vi "Read_Temp.vi"() -> ()   [LabVIEW 2013]
uses:
  <instrlib>/Mercury iXX/Public/Controls/Comms Transport Layer.ctl
  <instrlib>/Mercury iXX/Public/Controls/Serial Settings.ctl
  <instrlib>/Mercury iXX/Public/Controls/ISOBus Address.ctl
  <instrlib>/Mercury iXX/Public/Controls/Unit String.ctl
  <instrlib>/Mercury iXX/Public/Libraries/System/Open/Open System.vi
  <instrlib>/Mercury iXX/Public/Libraries/System/Read/Catalogue (Read).vi
  <instrlib>/Mercury iXX/Public/Libraries/Temperature/Open/Open Temperature Device.vi
  <instrlib>/Mercury iXX/Public/Libraries/Temperature/Signals/Read/Temperature (Read).vi
  <instrlib>/Mercury iXX/Mercury iXX.lvlib
  <instrlib>/Mercury iXX/Public/Libraries/System.lvlib
  <instrlib>/Mercury iXX/Public/Libraries/Temperature.lvlib
panel:
  in  "Read Interval (s)":sgl=1.0 min=0.25 max=1000 step=0.25 format="%.2f"
  in  "stop":bool
  out "Unit":T1
  out "Temperature":dbl
  out "error out":errorcluster
  in  "Device Identifier":string="MB1.T1:TEMP"
  in  "ISOBUS address":T2=-1 caption="ISOBUS address (-1)"
  out "Devices":string[](array[string])
  in  "Clear Previous Connections (False)":bool
  in  "ID Query (True)":bool
  in  "Serial Configuration":T3={"Baud Rate"=9600, "Parity"=0, "Data Bits"=8, "Stop Bits"=10, "Flow Control"=0} {"Flow Control" items=["None", "XON/XOFF", "RTS/CTS", "XON/XOFF & RTS/CTS", "DTR/DSR", "XON/XOFF & DTR/DSR"]; "Stop Bits" items=["1.0"=10, "2.0"=20]; "Data Bits" items=["7"=7, "8"=8]; "Parity" items=["None", "Odd", "Even"]; "Baud Rate" items=["300"=300, "600"=600, "1200"=1200, "2400"=2400, "4800"=4800, "9600"=9600, "19200"=19200]}
  in  "Comms Layer":T4
  in  "IP Address":string
  in  "VISA resource name":refnum<visa-resource-name>
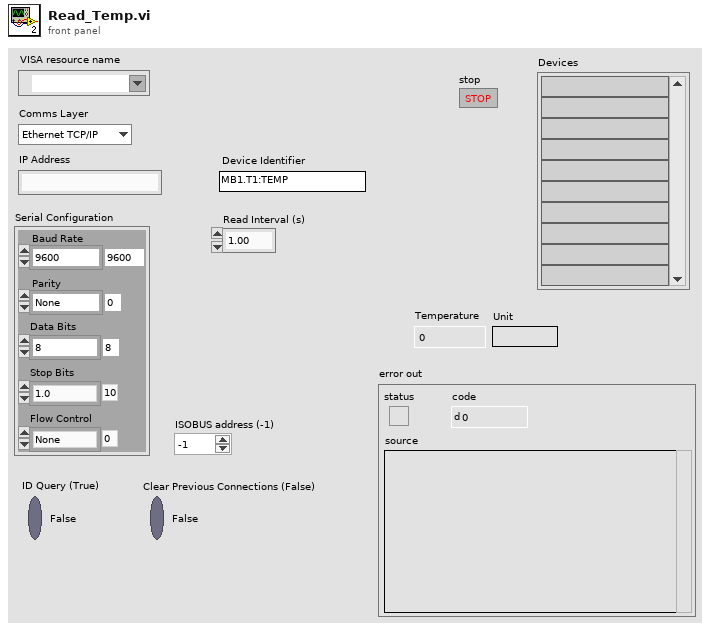
[diagram p1: front panel]
types:
  T1 = typedef "Mercury iXX.lvlib/Unit String.ctl" = string
  T2 = typedef "Mercury iXX.lvlib/ISOBus Address.ctl" = i32
  T3 = typedef "Mercury iXX.lvlib/Serial Settings.ctl" = cluster{"Baud Rate":u32, "Parity":u16, "Data Bits":u16, "Stop Bits":u16, "Flow Control":u16}
  T4 = typedef "Mercury iXX.lvlib/Comms Transport Layer.ctl" = enum16{"Ethernet TCP/IP", "USB", "ISOBus - RS-232", "GPIB"}
  T5 = typedef "Mercury iXX.lvlib/Mercury Reference.ctl" = cluster{"Comms":refnum<visa-resource-name>, "Device ID":string[], "Comms Layer":T4, "Command":string, "Query reference":T6}
  T6 = typedef "Mercury iXX.lvlib/Query Dynamic Reference.ctl" = refnum<vi>
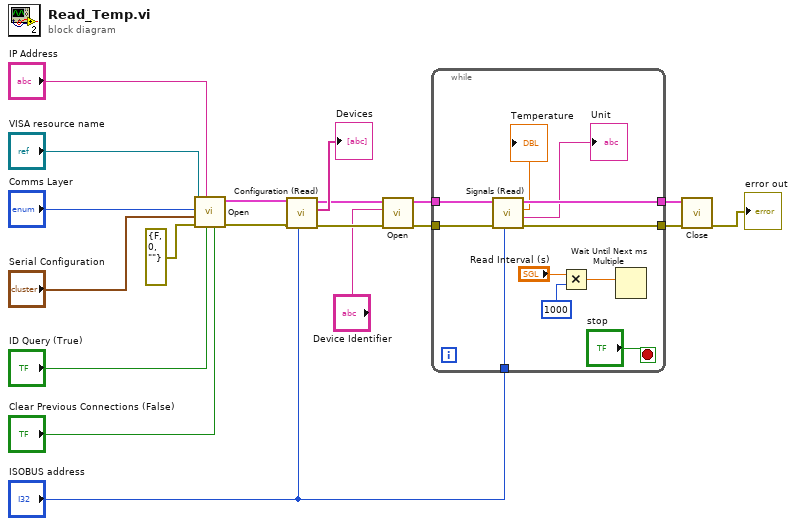
[diagram p0: block diagram]
diagram:
  n1 = call-poly <instrlib>:"Open.vi"("Clear Previous Connections (False)"="Clear Previous Connections (False)", "ID Query (True)"="ID Query (True)", "IP Address"="IP Address", "error in (no error)"=errorcluster {"status"=FALSE, "code"=0, "source"=""}, "Serial Configuration"="Serial Configuration", "Comms Layer"="Comms Layer", "VISA resource name"="VISA resource name") -> ("error out"=w11:errorcluster, "Mercury Reference Out"=w12:T5)  [unwired: 3 out]
  n2 = call-poly <instrlib>:"Configuration (Read).vi"("ISOBUS address"="ISOBUS address", "error in"=w11, "Mercury Reference In"=w12) -> ("error out"=w8:errorcluster, "Devices"=→"Devices":string[], "Mercury Reference Out"=w9:T5)  [unwired: 5 in, 1 out]
  n3 = call-poly <instrlib>:"Open.vi"("error in (no error)"=w8, "Device Identifier"="Device Identifier", "Mercury Reference In"=w9) -> ("error out"=w5:errorcluster, "Mercury Reference Out"=w6:T5)  [unwired: 7 in]
  n4 = while {
    tunnel: w6 -> [w30]
    tunnel: w5 -> [w29]
    tunnel: "ISOBUS address" -> [w28]
    tunnel: [w27] -> w3
    tunnel: [w26] -> w2
    stop <- "stop" stop-if-true
    n5 = call-poly <instrlib>:"Signals (Read).vi"("ISOBUS address"=w28, "error in"=w29, "Mercury Reference In"=w30) -> ("error out"=w27:errorcluster, "Unit"=→"Unit":T1, "Temperature"=→"Temperature":dbl, "Mercury Reference Out"=w26:T5)  [unwired: 4 in, 1 out]
    n6 = Multiply(x="Read Interval (s)", y=u32 1000 ("millisecond multiple")) -> (x*y=w20:sgl)
    n7 = Wait Until Next ms Multiple(millisecond multiple=w20) -> ()  [unwired: 1 out]
  }
  n8 = call <instrlib>:"Close.vi"("error in (no error)"=w3, "Mercury Reference"=w2) -> ("error out"=→"error out":errorcluster)  [unwired: 9 in]
